vi "Imaq ReadFile.vi"() -> ()   [LabVIEW 2015]
panel:
  out "Image":T1(plugin-control)
  in  "File Path":path
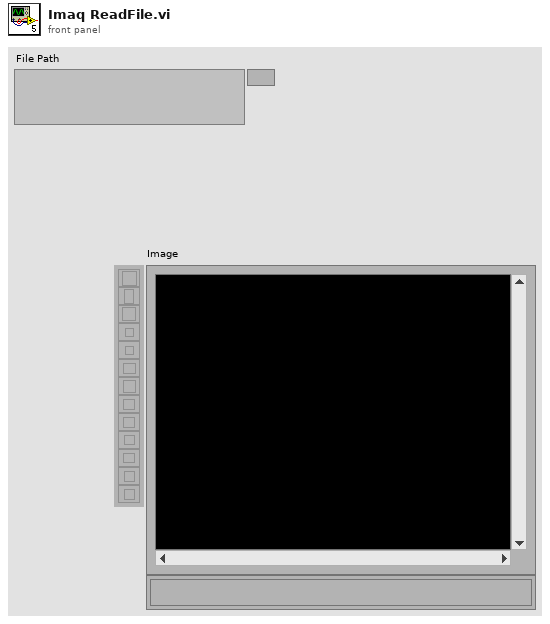
[diagram p1: front panel]
types:
  T1 = typedef "IMAQ Image.ctl" = refnum<image>
  T2 = typedef "Image Type" = u32
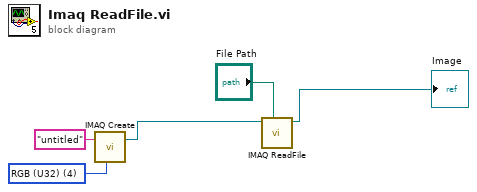
[diagram p0: block diagram]
diagram:
  w4 = T2 4 items=["Grayscale (U8)", "Grayscale (I16)", "Grayscale (SGL)", "Complex (CSG)", "RGB (U32)", "HSL (U32)", "RGB (U64)", "Grayscale (U16)"] ("Image Type")
  n1 = call "IMAQ Create"("Image Name"="untitled", "Image Type"=w4) -> ("New Image"=w3:T1)  [unwired: 3 in, 1 out]
  n2 = call "IMAQ ReadFile"("File Path"="File Path", "Image"=w3) -> ("Image Out"=→"Image":T1)  [unwired: 5 in, 4 out]
